vi "glue_dispenser.vi"() -> ()   [LabVIEW 2016]
uses:
  <vilib>/LabVIEW Interface for Arduino/Type Defs/Pin Mode.ctl
  <vilib>/Utility/file.llb/Read Delimited Spreadsheet (DBL).vi
  <vilib>/LabVIEW Interface for Arduino/LabVIEW Interface for Arduino.lvlib
panel:
  in  "File to be processed":path=path "C:/Users/Aerotech/Documents/BNL_ThermomechanicalStave/1_ModulePlacement/1_GluePatterning/LabVIEW_gluepattern_array.csv"
  in  "Axis Speeds":T1
  in  "Go to \ncoordinates":T2
  out "DX [s]":dbl format="%#_2g"
  out "DY [s]":dbl format="%#_2g"
  in  "Module width [mm]":dbl
  in  "Module length [mm]":dbl
  out "INPUT":bool[][](array[boolean])
  out "Row":i32
  out "Column":i32
  in  "Duration of glue \ndispensing [s]":dbl
  out "error out":errorcluster
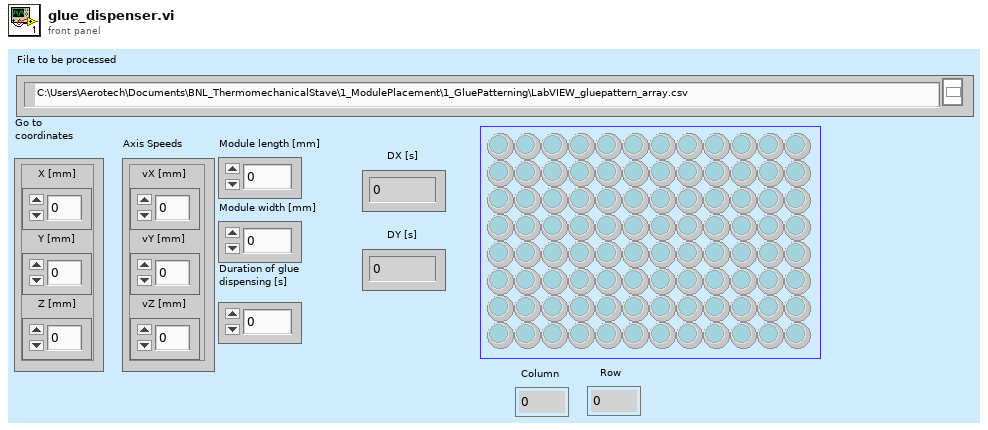
[diagram p1: front panel]
types:
  T1 = cluster{"vX [mm]":dbl, "vY [mm]":dbl, "vZ [mm] ":dbl}
  T2 = cluster{"X [mm]":dbl, "Y [mm]":dbl, "Z [mm] ":dbl}
  T3 = typedef "LabVIEW Interface for Arduino.lvlib/Pin Mode.ctl" = enum8{"Input", "Output"}
  T4 = typedef "LabVIEW Interface for Arduino.lvlib/Arduino Resource.ctl" = cluster{"VISA resource":refnum<visa-resource-name>, "Board Type":T5, "Connection Type":enum8{"USB / Serial"}, "Bytes Per Packet (15)":u8}
  T5 = typedef "LabVIEW Interface for Arduino.lvlib/Board Type.ctl" = enum16{"Uno", "Dimuelanove w/Atmega 328", "Mega 2560"}
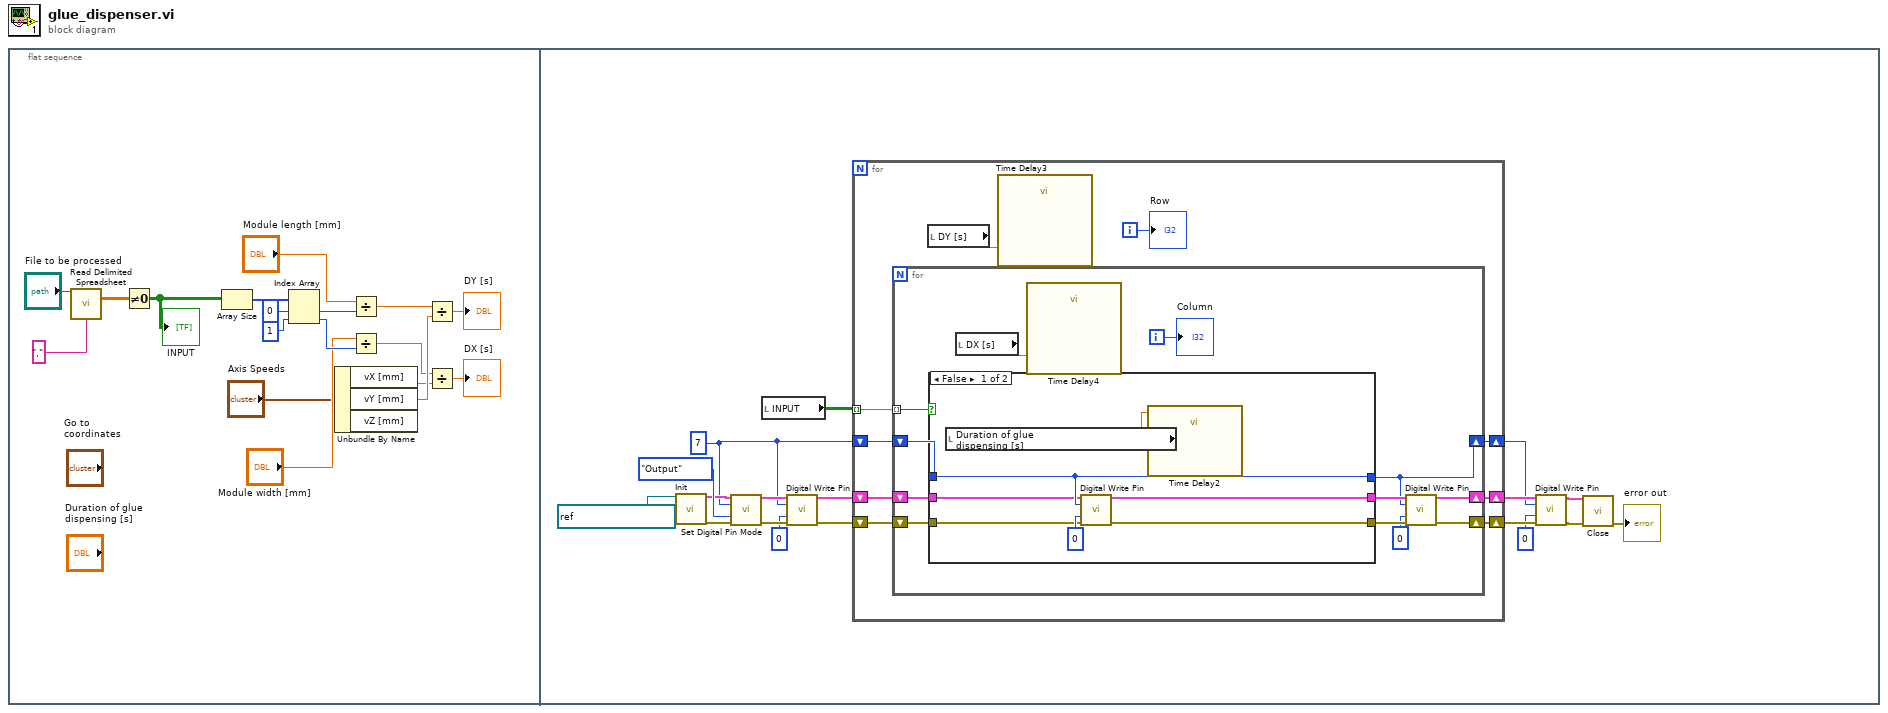
[diagram p0: block diagram]
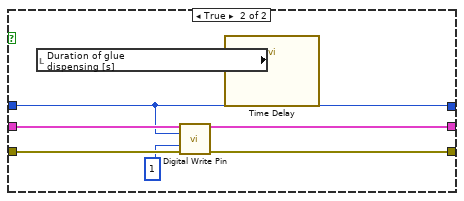
[diagram p2: hidden frame]
diagram:
  n1 = flat-sequence {
    frame #0 {
      n2 = call-poly <vilib>:"Read Delimited Spreadsheet.vi"("file path (dialog if empty)"="File to be processed", "delimiter (\\t)"="," ("delimiter (\\t)")) -> ("all rows"=w17:dbl[][])  [unwired: 8 in, 5 out]
      n3 = Not Equal To 0?(x=w17) -> (x != 0?=w16:bool[][])
      "INPUT" <- w16
      n4 = Array Size(array=w16) -> (size(s)=w15:i32[])
      n5 = Index Array(array=w15, index #1=0 ("index"), index #2=1 ("index")) -> (element #1=w11:i32, element #2=w10:i32)
      n6 = Unbundle By Name("Axis Speeds") -> ("vX [mm]"=w5:dbl, "vY [mm]"=w7:dbl)  [unwired: 1 out]
      n7 = Divide(x="Module length [mm]", y=w11) -> (x/y=w8:dbl)
      n8 = Divide(x="Module width [mm]", y=w10) -> (x/y=w4:dbl)
      n9 = Divide(x=w8, y=w7) -> (x/y=→"DY [s]":dbl)
      n10 = Divide(x=w4, y=w5) -> (x/y=→"DX [s]":dbl)
    }
    frame #1 {
      w21 = u8 7 ("Digital I/O Pin")
      n11 = call <vilib>:"Init.vi"("VISA resource"=refnum<visa-resource-name> "ASRL2::INSTR") -> ("Arduino Resource"=w28:T4, "error out"=w30:errorcluster)  [unwired: 17 in]
      n12 = call <vilib>:"Set Digital Pin Mode.vi"("Arduino Resource"=w28, "Digital I/O Pin"=w21, "Pin Mode (Input)"=Pin_Mode."Output", "error in"=w30) -> ("Arduino Resource"=w26:T4, "error out"=w25:errorcluster)  [unwired: 10 in]
      n13 = local read "INPUT"() -> (w19:bool[][])
      n14 = call <vilib>:"Digital Write Pin.vi"("Arduino Resource"=w26, "Digital I/O Pin (0)"=w21, "Value (0)"=u8 0, "error in"=w25) -> ("Arduino Resource"=w24:T4, "error out"=w23:errorcluster)  [unwired: 10 in]
      n15 = for {
        shift-right: [w41] -> w34
        shift-left: w24 -> [w45]
        shift-right: [w42] -> w33
        shift-left: w23 -> [w44]
        shift-right: [w40] -> w20
        shift-left: w21 -> [w43]
        tunnel: w19 -> [w38] mode=indexing
        i -> [w37]
        n16 = for {
          shift-right: [w51] -> w41
          shift-left: w45 -> [w57]
          shift-right: [w53] -> w42
          shift-left: w44 -> [w56]
          shift-right: [w50] -> w40
          shift-left: w43 -> [w55]
          tunnel: w38 -> [w47] mode=indexing
          i -> [w46]
          n17 = case shown="False" w47 {
            tunnel: w57 -> [w62 w71]
            tunnel: w56 -> [w60 w70]
            tunnel: w55 -> [w63 w67]
            tunnel: [w59 w69] -> w54
            tunnel: [w61 w68] -> w52
            tunnel: [w63 w67] -> w50
            frame False {
              n18 = local read "Duration of glue \ndispensing [s]"() -> (w58:dbl)
              n19 = call <vilib>:"Digital Write Pin.vi"("Arduino Resource"=w62, "Digital I/O Pin (0)"=w63, "Value (0)"=u8 0, "error in"=w60) -> ("Arduino Resource"=w61:T4, "error out"=w59:errorcluster)  [unwired: 10 in]
              n20 = call "Time Delay2"("Delay Time (s)"=w58) -> ()  [unwired: 10 in, 1 out]
            }
            frame True {
              n21 = local read "Duration of glue \ndispensing [s]"() -> (w65:dbl)
              n22 = call <vilib>:"Digital Write Pin.vi"("Arduino Resource"=w71, "Digital I/O Pin (0)"=w67, "Value (0)"=u8 1, "error in"=w70) -> ("Arduino Resource"=w68:T4, "error out"=w69:errorcluster)  [unwired: 10 in]
              n23 = call "Time Delay"("Delay Time (s)"=w65) -> ()  [unwired: 10 in, 1 out]
            }
          }
          n24 = local read "DX [s]"() -> (w48:dbl)
          n25 = call "Time Delay4"("Delay Time (s)"=w48) -> ()  [unwired: 10 in, 1 out]
          n26 = call <vilib>:"Digital Write Pin.vi"("Arduino Resource"=w52, "Digital I/O Pin (0)"=w50, "Value (0)"=u8 0, "error in"=w54) -> ("Arduino Resource"=w51:T4, "error out"=w53:errorcluster)  [unwired: 10 in]
          "Column" <- w46
        }
        n27 = local read "DY [s]"() -> (w39:dbl)
        n28 = call "Time Delay3"("Delay Time (s)"=w39) -> ()  [unwired: 10 in, 1 out]
        "Row" <- w37
      }
      n29 = call <vilib>:"Digital Write Pin.vi"("Arduino Resource"=w34, "Digital I/O Pin (0)"=w20, "Value (0)"=u8 0, "error in"=w33) -> ("Arduino Resource"=w35:T4, "error out"=w36:errorcluster)  [unwired: 10 in]
      n30 = call <vilib>:"Close.vi"("Arduino Resource"=w35, "error in"=w36) -> ("error out"=→"error out":errorcluster)  [unwired: 13 in]
    }
  }
